vi "fit maj axis data to exponential decay.vi"(7 "hrs":bool=TRUE, 10 "length":i32=2147483647, 11 "extracted data":T1[](array[typedef])) -> (2 "graphs":cluster{dbl[], dbl[]}[](array[cluster]), 3 "lifetime":dbl, 5 "Q":dbl)   [LabVIEW 2020]
uses:
  typedefs/reading.ctl
  typedefs/readingType.ctl
  <vilib>/Analysis/NI_AALPro.lvlib
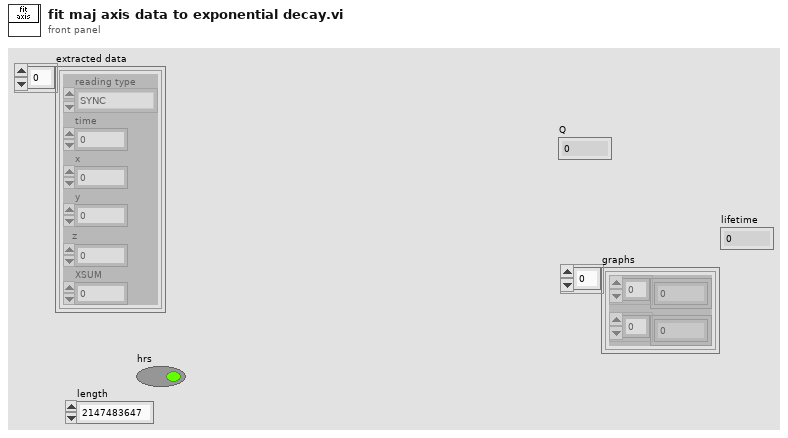
[diagram p1: front panel]
types:
  T1 = typedef "reading.ctl" = cluster{"reading type":T2, "time":fxp<+,48,48>, "x":sgl, "y":sgl, "z":sgl, "XSUM":u8}
  T2 = typedef "readingType.ctl" = enum8{"SYNC", "DETVAL", "COILI", "MAGVEC", "ACCVEC", "CROSSING", "MAGVEC0", "MAGVEC1", "MAGVEC2", "MAGVEC3", "MAGVEC4", "MAGVEC5", "MAGVEC6", "MAGVEC7"}
  T3 = cluster{"amp min":dbl, "amp max":dbl, "damping min":dbl, "damping max":dbl, "offset min":dbl, "offset max":dbl}
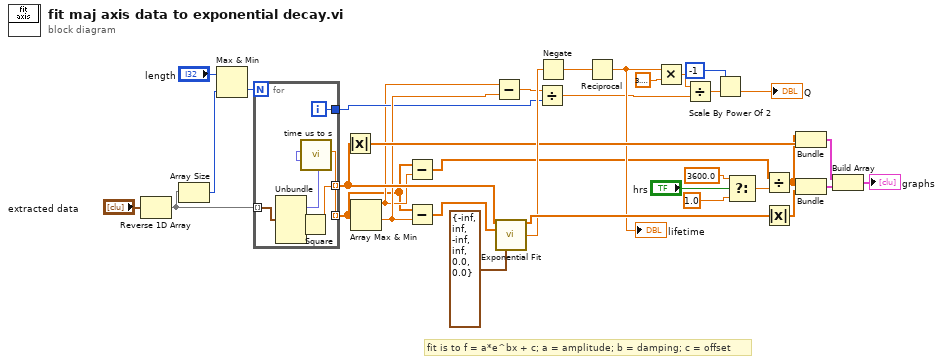
[diagram p0: block diagram]
diagram:
  # "fit is to f = a*e^bx + c; a = amplitude; b = damping; c = offset"
  n1 = Reverse 1D Array(array="extracted data") -> (reversed array=w33:T1[])
  n2 = Array Size(array=w33) -> (size(s)=w32:i32)
  n3 = Max & Min(x="length", y=w32) -> (min(x,y)=w30:i32)  [unwired: 1 out]
  n4 = for {
    N: w30 -> [_]
    tunnel: w33 -> [w40] mode=indexing
    tunnel: [w37] -> w4 mode=indexing
    tunnel: [w35] -> w29 mode=indexing
    tunnel: [w39] -> w11
    i -> [w39]
    n5 = Unbundle(w40) -> ("time"=w38:fxp<+,48,48>, "y"=w36:sgl)  [unwired: 4 out]
    n6 = Square(x=w36) -> (x^2=w35:sgl)
    n7 = call "time us to s.vi"("time (us)"=w38) -> ("time (s)"=w37:dbl)  [unwired: 10 in]
  }
  n8 = Absolute Value(x=w29) -> (abs(x)=w20:sgl[])
  n9 = Array Max & Min(array=w4) -> (max value=w5:dbl, min value=w13:dbl)  [unwired: 2 out]
  n10 = Subtract(x=w4, y=w5) -> (x-y=w3:dbl[])
  n11 = Subtract(x=w4, y=w13) -> (x-y=w19:dbl[])
  n12 = Subtract(x=w5, y=w13) -> (x-y=w12:dbl)
  n13 = call <vilib>:"Exponential Fit.vi"("Y"=w29, "X"=w19, "parameter bounds"=T3 {"amp min"=-inf, "amp max"=inf, "damping min"=-inf, "damping max"=inf, "offset min"=0.0, "offset max"=0.0}) -> ("Best Exponential Fit"=w26:dbl[], "damping"=w25:dbl)  [unwired: 7 in, 4 out]
  n14 = Divide(x=w12, y=w11) -> (x/y=w7:dbl)
  n15 = Negate(x=w25) -> (-x=w24:dbl)
  n16 = Reciprocal(x=w24) -> (1/x=w9:dbl)
  "lifetime" <- w9
  n17 = Multiply(x=w9, y=3.141592653589793) -> (x*y=w8:dbl)
  n18 = Divide(x=w8, y=w7) -> (x/y=w6:dbl)
  n19 = Scale By Power Of 2(n=i16 -1, x=w6) -> (x*2^n=→"Q":dbl)
  n20 = Select(t=3600.0, s="hrs", f=1.0 ("t")) -> (s? t:f=w17:dbl)
  n21 = Divide(x=w3, y=w17) -> (x/y=w14:dbl[])
  n22 = Absolute Value(x=w26) -> (abs(x)=w21:dbl[])
  n23 = Bundle(w14, w20) -> (w28:cluster{dbl[], sgl[]})  [unwired: 1 in]
  n24 = Bundle(w14, w21) -> (w23:cluster{dbl[], dbl[]})  [unwired: 1 in]
  n25 = Build Array(w28, w23) -> (→"graphs":cluster{dbl[], dbl[]}[])
